vi "LWXPS_ZygoADCDiagnosticStatusGet.vi"(0 "XPS Reference IN":refnum<k24>, 5 "Axis":i32, 7 "ADC mux number":i32, 11 "LabVIEW error IN":errorcluster) -> (4 "XPS Reference OUT":refnum<k24>, 6 "Returned error code":i32, 8 "ADC diagnostic status":string, 10 "XPS Error String":string, 15 "LabVIEW error OUT":errorcluster)   [LabVIEW 2014]
uses:
  D:/XPSQ8_LabView_Library/Development/Source/Dll/Newport.XPS.CommandInterface.dll
  Dll/Newport.XPS.CommandInterface.dll
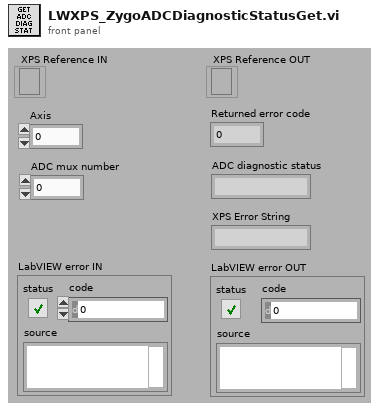
[diagram p1: front panel]
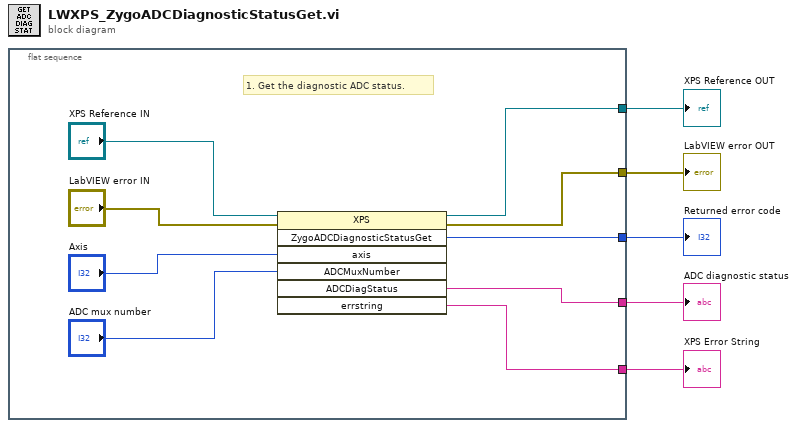
[diagram p0: block diagram]
diagram:
  n1 = flat-sequence {
    tunnel: [w12] -> w5
    tunnel: [w10] -> w4
    tunnel: [w13] -> w3
    tunnel: [w9] -> w2
    tunnel: [w8] -> w1
    frame #0 {
      # "1. Get the diagnostic ADC status."
      n2 = invoke class="XPS" method="ZygoADCDiagnosticStatusGet"(reference="XPS Reference IN", error in="LabVIEW error IN", "axis"="Axis", "ADCMuxNumber"="ADC mux number") -> (reference out=w12:refnum<k24>, error out=w10:errorcluster, "ZygoADCDiagnosticStatusGet"=w13:i32, "ADCDiagStatus"=w9:string, "errstring"=w8:string)  [unwired: 3 in, 2 out]
    }
  }
  "XPS Error String" <- w1
  "XPS Reference OUT" <- w5
  "LabVIEW error OUT" <- w4
  "Returned error code" <- w3
  "ADC diagnostic status" <- w2
